vi "case_struct.vi"() -> ()   [LabVIEW 2020]
uses:
  <vilib>/ErrorRing/Error Ring.xnode
panel:
  out "String 2":string
  in  "String":string
  out "Numeric 2":dbl
  in  "Numeric":u8
  out "Boolean 2":bool
  in  "Boolean":bool
  in  "stop":bool
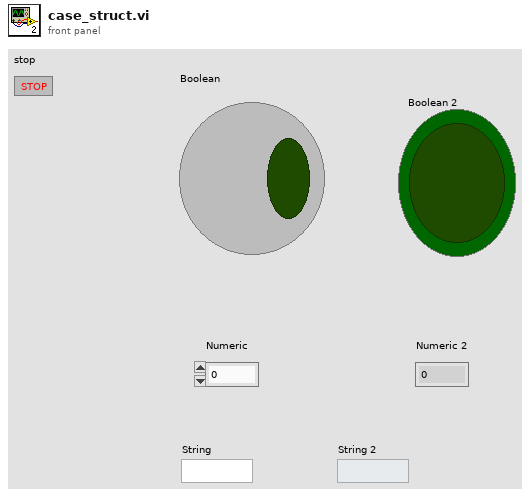
[diagram p1: front panel]
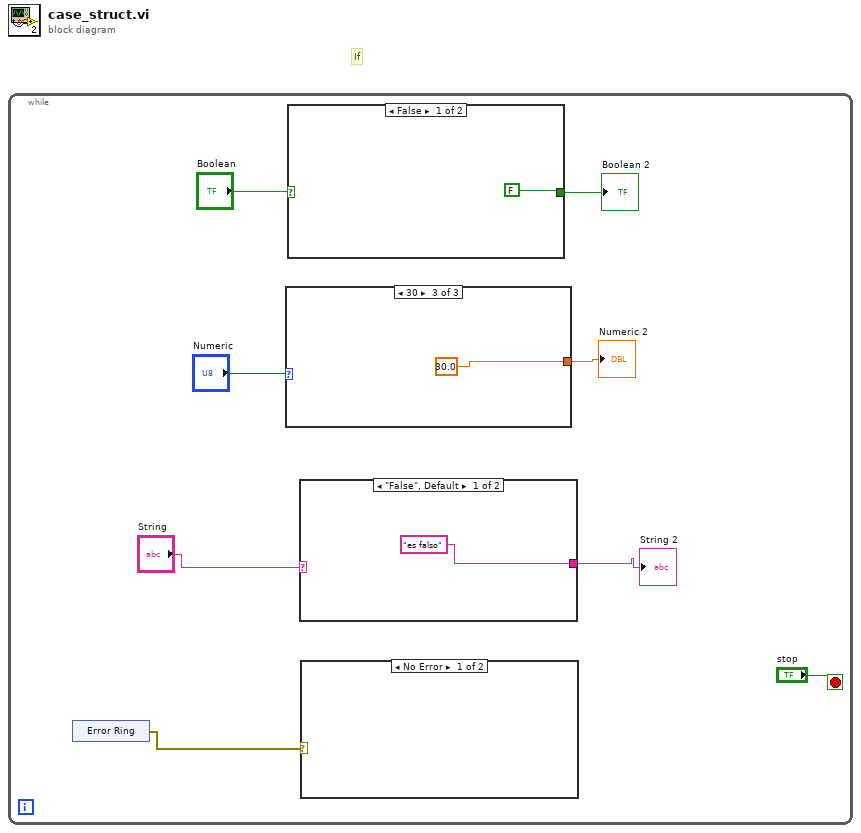
[diagram p0: block diagram]
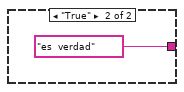
[diagram p3: hidden frame]
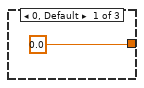
[diagram p4: hidden frame]
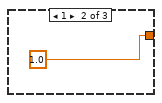
[diagram p5: hidden frame]
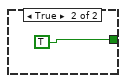
[diagram p6: hidden frame]
diagram:
  # "If"
  n1 = while {
    stop <- "stop" stop-if-true
    n2 = xnode "Error Ring"() -> ("error out"=w1:errorcluster)
    n3 = case shown="30" "Numeric" {
      tunnel: [0.0 1.0 30.0] -> w4
      frame 0, Default {
      }
      frame 1 {
      }
      frame 30 {
      }
    }
    "Numeric 2" <- w4
    n4 = case shown="False" "Boolean" {
      tunnel: [FALSE TRUE] -> w6
      frame False {
      }
      frame True {
      }
    }
    "Boolean 2" <- w6
    n5 = case shown="\"False\", Default" "String" {
      tunnel: ["es falso" "es  verdad"] -> w2
      frame "False", Default {
      }
      frame "True" {
      }
    }
    "String 2" <- w2
    n6 = case shown="No Error" w1 {
      frame No Error {
      }
      frame Error {
      }
    }
  }
